vi "BEditor-Localization.vi"(7 "Reference":variant, 8 "Error in":errorcluster caption="Error in (no error)", 9 "Option":variant, 11 "Entry":string) -> (0 "Error out":errorcluster)   [LabVIEW 2017, in "csmdoc.lvlib"]
uses:
  csmdoc.lvlib
  _Typedef/DocElement.ctl
  Communicable State Machine.lvlib
  _Shared/CSM Shared.lvlib
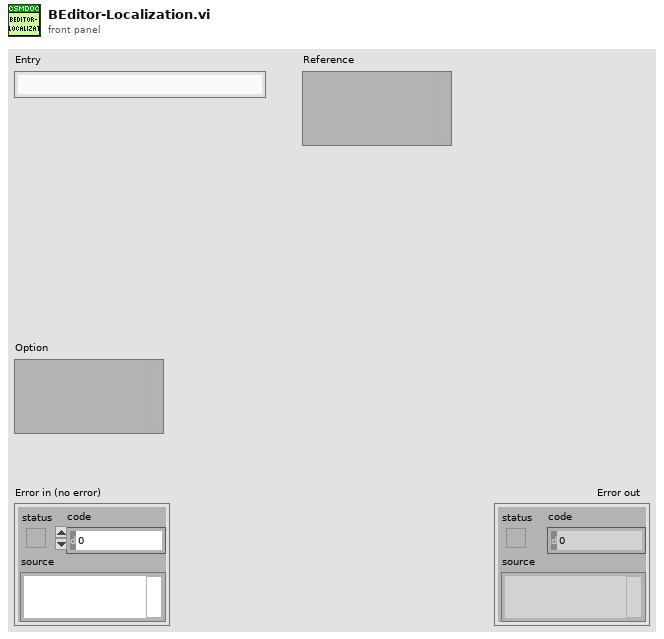
[diagram p1: front panel]
types:
  T1 = typedef "csmdoc.lvlib/DocElement.ctl" = cluster{"ID":string, "Content":string[], "SubIDs":string[], "Path":string[]}
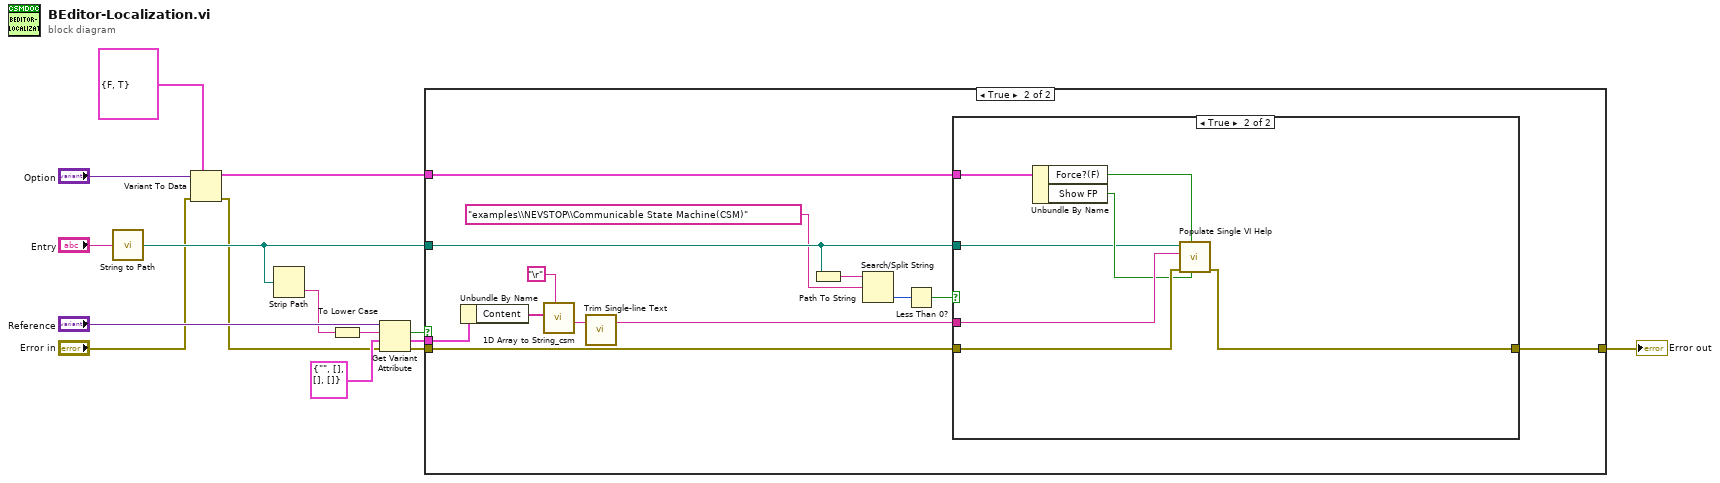
[diagram p0: block diagram]
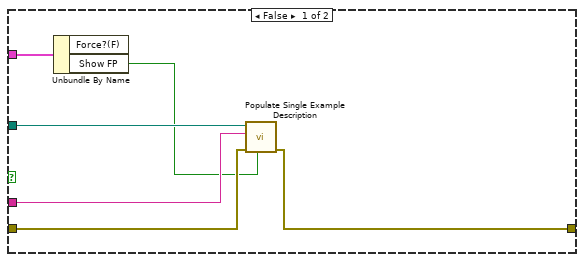
[diagram p3: hidden frame]
diagram:
  n1 = call "String to Path.vi"("String"="Entry") -> ("Path"=w6:path)
  n2 = Variant To Data(error in="Error in", type=cluster{"Force?(F)":bool, "Show FP":bool} {"Force?(F)"=FALSE, "Show FP"=TRUE}, Variant="Option") -> (data=w1:cluster{"Force?(F)":bool, "Show FP":bool}, error out=w2:errorcluster)
  n3 = Strip Path(path=w6) -> (name=w13:string)  [unwired: 1 out]
  n4 = To Lower Case(string=w13) -> (all lower case string=w9:string)
  n5 = Get Variant Attribute(Variant="Reference", name=w9, default value (empty Variant)=T1 {"ID"="", "Content"=[], "SubIDs"=[], "Path"=[]} ("Cluster"), error in=w2) -> (found=w12:bool, value=w10:T1, error out=w11:errorcluster)  [unwired: 1 out]
  n6 = case shown="True" w12 {
    tunnel: w6 -> [_ w21]
    tunnel: w11 -> [w16 w29]
    tunnel: [w16 w28] -> w7
    tunnel: w10 -> [_ w24]
    tunnel: w1 -> [_ w22]
    frame False {
    }
    frame True {
      n7 = Unbundle By Name(w24) -> ("Content"=w27:string[])
      n8 = call "1D Array to String_csm.vi"("delimiter (Tab)"="\r", "Array of Strings"=w27) -> ("delimited string"=w25:string)  [unwired: 9 in]
      n9 = call "Trim Single-line Text.vi"("single-line text"=w25) -> ("trimed text"=w23:string)  [unwired: 2 in]
      n10 = Path To String(path=w21) -> (string=w20:string)
      n11 = Search/Split String(string=w20, search string/char (-)="examples\\NEVSTOP\\Communicable State Machine(CSM)") -> (offset of match=w18:i32)  [unwired: 1 in, 2 out]
      n12 = Less Than 0?(x=w18) -> (x < 0?=w17:bool)
      n13 = case shown="True" w17 {
        tunnel: w29 -> [w34 w42]
        tunnel: [w33 w41] -> w28
        tunnel: w23 -> [w32 w40]
        tunnel: w22 -> [w31 w39]
        tunnel: w21 -> [w35 w36]
        frame False {
          n14 = Unbundle By Name(w31) -> ("Show FP"=w30:bool)  [unwired: 1 out]
          n15 = call "Populate Single Example Description.vi"("Show FP"=w30, "error in (no error)"=w34, "VI Description"=w32, "Path"=w35) -> ("error out"=w33:errorcluster)  [unwired: 7 in]
        }
        frame True {
          n16 = Unbundle By Name(w39) -> ("Force?(F)"=w38:bool, "Show FP"=w37:bool)
          n17 = call "Populate Single VI Help.vi"("Show FP"=w37, "Force?(F)"=w38, "error in (no error)"=w42, "VI Description"=w40, "Path"=w36) -> ("error out"=w41:errorcluster)  [unwired: 6 in]
        }
      }
    }
  }
  "Error out" <- w7
